vi "i2c_osd_cmd_write.vi"(5 "COM":bool, 7 "VISA name":refnum<visa-resource-name>, 9 "data":u8[](array[numeric]), 10 "byDataLen":u8, 11 "vdcmd_info_osd_t":T1) -> (3 "return":i32)   [LabVIEW 2016]
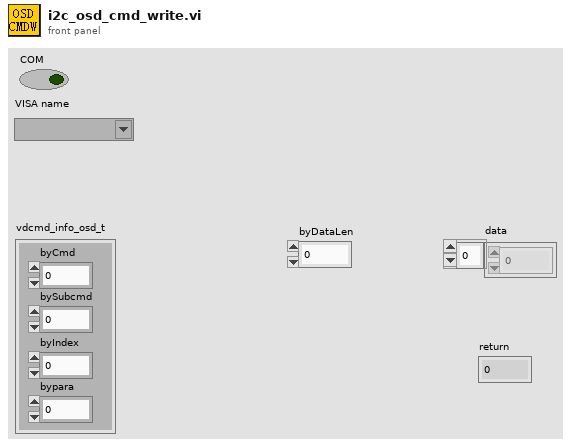
[diagram p1: front panel]
types:
  T1 = cluster{"byCmd":u8, "bySubcmd":u8, "byIndex":u8, "bypara":u8}
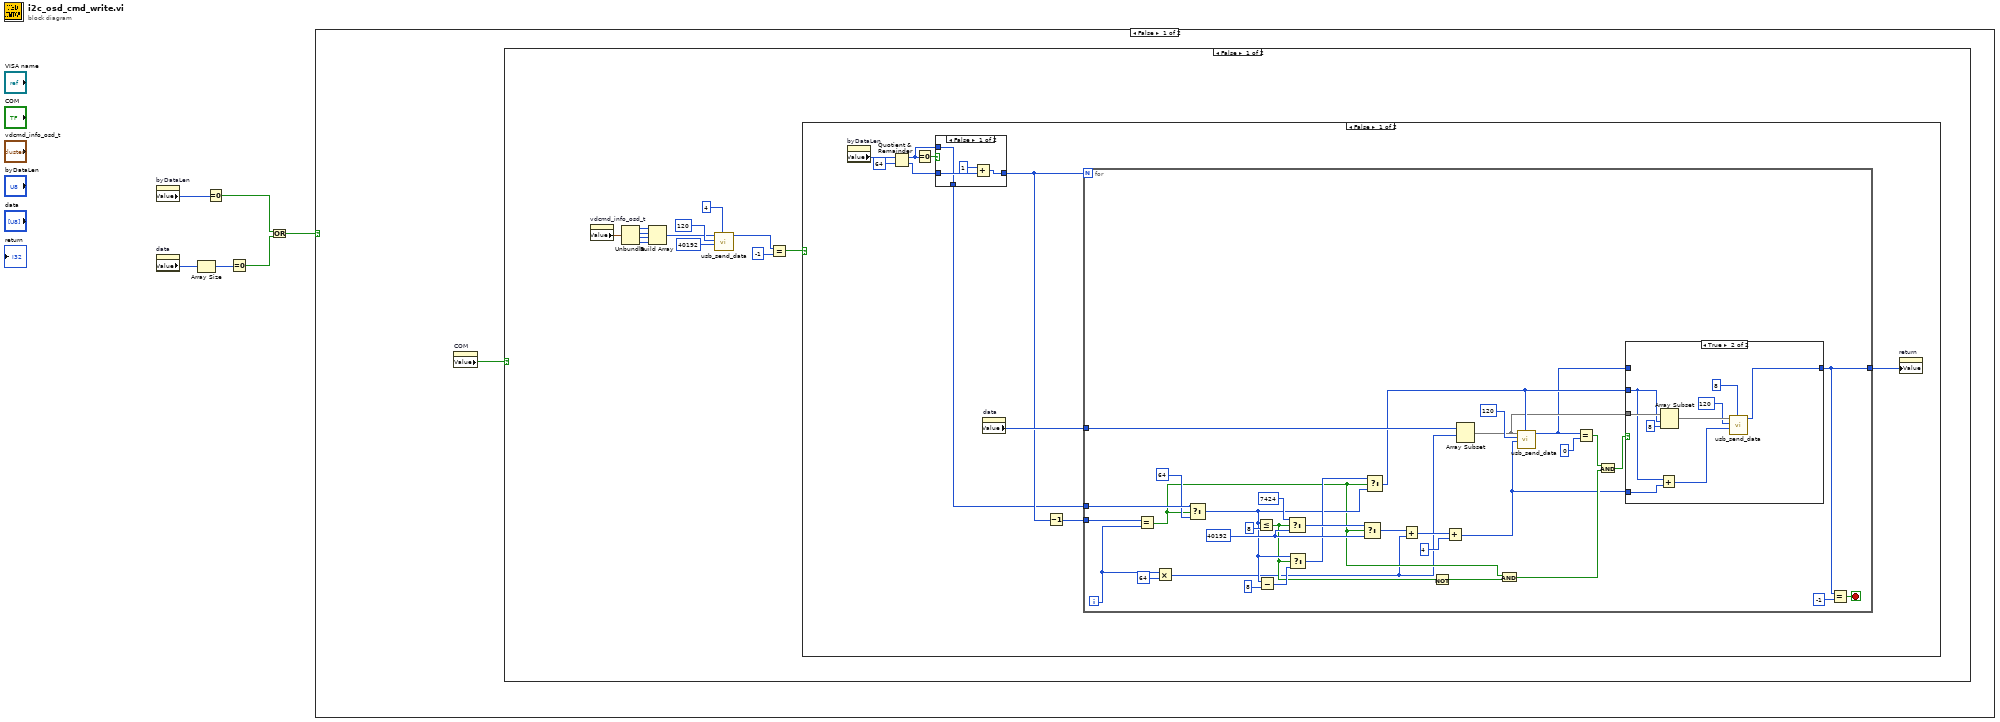
[diagram p0: block diagram]
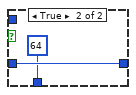
[diagram p3: hidden frame]
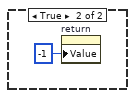
[diagram p4: hidden frame]
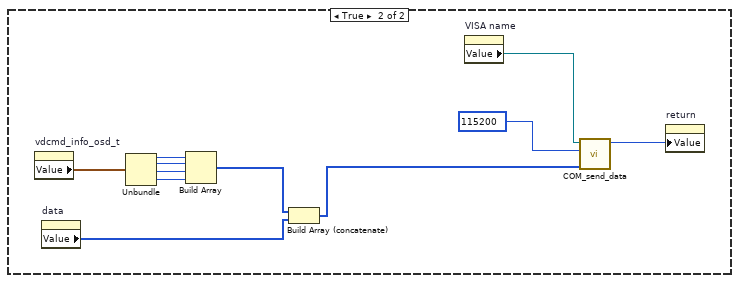
[diagram p5: hidden frame]
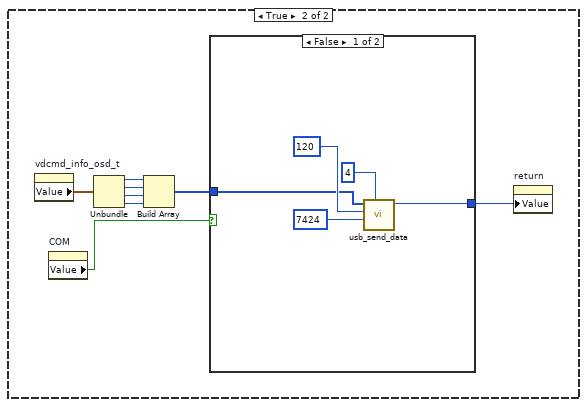
[diagram p6: hidden frame]
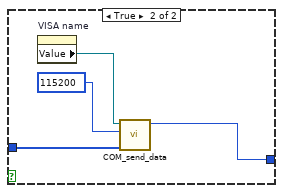
[diagram p7: hidden frame]
diagram:
  n1 = property on="byDataLen" class="DigNum (strict)"() -> ("Value"=w6:u8)  [unwired: 2 in, 2 out]
  n2 = property on="data" class="Arr (strict)"() -> ("Value"=w5:u8[])  [unwired: 2 in, 2 out]
  n3 = Array Size(array=w5) -> (size(s)=w4:i32)
  n4 = Equal To 0?(x=w6) -> (x = 0?=w2:bool)
  n5 = Equal To 0?(x=w4) -> (x = 0?=w3:bool)
  n6 = Or(x=w2, y=w3) -> (x .or. y?=w1:bool)
  n7 = case shown="False" w1 {
    frame False {
      n8 = property on="COM" class="Bool (strict)"() -> ("Value"=w7:bool)  [unwired: 2 in, 2 out]
      n9 = case shown="False" w7 {
        frame False {
          n10 = property on="vdcmd_info_osd_t" class="Clust (strict)"() -> ("Value"=w16:T1)  [unwired: 2 in, 2 out]
          n11 = Unbundle(w16) -> ("byCmd"=w15:u8, "bySubcmd"=w14:u8, "byIndex"=w13:u8, "bypara"=w12:u8)
          n12 = Build Array(w15, w14, w13, w12) -> (w11:u8[])
          n13 = call "usb_send_data.vi"("byVdCmdHeaderLen"=u16 4, "I2C_VD_BUFFER_RW"=u16 40192, "I2C_SLAVE_ID"=u8 120, "data"=w11) -> ("return"=w10:i32)  [unwired: 6 in, 1 out]
          n14 = Equal?(x=w10, y=-1) -> (x = y?=w8:bool)
          n15 = case shown="False" w8 {
            frame False {
              n16 = property on="byDataLen" class="DigNum (strict)"() -> ("Value"=w29:u8)  [unwired: 2 in, 2 out]
              n17 = Quotient & Remainder(x=w29, y=u8 64) -> (x-y*floor(x/y)=w23:u8, floor(x/y)=w26:u8)
              n18 = Equal To 0?(x=w23) -> (x = 0?=w27:bool)
              n19 = case shown="False" w27 {
                tunnel: w26 -> [w76 w78]
                tunnel: [w75 w78] -> w24
                tunnel: w23 -> [w73 _]
                tunnel: [w73 u8 64] -> w22
                frame False {
                  n20 = Add(x=u8 1, y=w76) -> (x+y=w75:u8)
                }
                frame True {
                }
              }
              n21 = property on="data" class="Arr (strict)"() -> ("Value"=w25:u8[])  [unwired: 2 in, 2 out]
              n22 = Decrement(x=w24) -> (x-1=w21:u8)
              n23 = for {
                N: w24 -> [_]
                tunnel: w25 -> [w60]
                tunnel: w21 -> [w62]
                tunnel: w22 -> [w58]
                tunnel: [w31] -> w20
                i -> [w59]
                stop <- w32 stop-if-true
                w47 = u16 40192 ("y")
                n24 = Equal?(x=w62, y=w59) -> (x = y?=w42:bool)
                n25 = Multiply(x=w59, y=64) -> (x*y=w30:i32)
                n26 = Select(t=w58, s=w42, f=u8 64) -> (s? t:f=w45:u8)
                n27 = Less Or Equal?(x=w45, y=u8 8) -> (x <= y?=w43:bool)
                n28 = Subtract(x=w45, y=u8 8) -> (x-y=w53:u8)
                n29 = Select(t=u16 7424 ("y"), s=w43, f=w47) -> (s? t:f=w48:u16)
                n30 = Select(t=w45, s=w43, f=w53) -> (s? t:f=w46:u8)
                n31 = Select(t=w48, s=w42, f=w47) -> (s? t:f=w49:u16)
                n32 = Select(t=w46, s=w42, f=w45) -> (s? t:f=w38:u8)
                n33 = Add(x=w49, y=w30) -> (x+y=w52:i32)
                n34 = Not(x=w43) -> (.not. x?=w41:bool)
                n35 = Add(x=w52, y=u16 4) -> (x+y=w36:i32)
                n36 = Array Subset(array=w60, index=w30) -> (w37:u8[])  [unwired: 1 in]
                n37 = And(x=w42, y=w41) -> (x .and. y?=w40:bool)
                n38 = call "usb_send_data.vi"("byVdCmdHeaderLen"=w38, "I2C_VD_BUFFER_RW"=w36, "I2C_SLAVE_ID"=u8 120, "data"=w37) -> ("return"=w34:i32)  [unwired: 6 in, 1 out]
                n39 = Equal?(x=w34, y=0) -> (x = y?=w35:bool)
                n40 = And(x=w35, y=w40) -> (x .and. y?=w39:bool)
                n41 = case shown="True" w39 {
                  tunnel: w38 -> [_ w67]
                  tunnel: w37 -> [_ w72]
                  tunnel: w36 -> [_ w68]
                  tunnel: w34 -> [w63 _]
                  tunnel: [w63 w65] -> w31
                  frame False {
                  }
                  frame True {
                    n42 = Add(x=w67, y=w68) -> (x+y=w66:i32)
                    n43 = Array Subset(array=w72, index=w67, length=8) -> (w70:u8[])
                    n44 = call "usb_send_data.vi"("byVdCmdHeaderLen"=u16 8, "I2C_VD_BUFFER_RW"=w66, "I2C_SLAVE_ID"=u8 120, "data"=w70) -> ("return"=w65:i32)  [unwired: 6 in, 1 out]
                  }
                }
                n45 = Equal?(x=w31, y=-1) -> (x = y?=w32:bool)
              }
              n46 = property on="return" class="DigNum (strict)"("Value"=w20) -> ()  [unwired: 2 in, 2 out]
            }
            frame True {
              n47 = property on="return" class="DigNum (strict)"("Value"=-1 ("return")) -> ()  [unwired: 2 in, 2 out]
            }
          }
        }
        frame True {
          n48 = property on="vdcmd_info_osd_t" class="Clust (strict)"() -> ("Value"=w88:T1)  [unwired: 2 in, 2 out]
          n49 = property on="data" class="Arr (strict)"() -> ("Value"=w82:u8[])  [unwired: 2 in, 2 out]
          n50 = Unbundle(w88) -> ("byCmd"=w87:u8, "bySubcmd"=w86:u8, "byIndex"=w85:u8, "bypara"=w84:u8)
          n51 = Build Array(w87, w86, w85, w84) -> (w83:u8[])
          n52 = Build Array (concatenate)(w83, w82) -> (w81:u8[])
          n53 = property on="VISA name" class="VISAName"() -> ("Value"=w90:refnum<visa-resource-name>)  [unwired: 2 in, 2 out]
          n54 = call "COM_send_data.vi"("data"=w81, "baud rate (9600)"=u32 115200, "VISA name"=w90) -> ("return"=w80:i32)  [unwired: 8 in]
          n55 = property on="return" class="DigNum (strict)"("Value"=w80) -> ()  [unwired: 2 in, 2 out]
        }
      }
    }
    frame True {
      n56 = property on="vdcmd_info_osd_t" class="Clust (strict)"() -> ("Value"=w98:T1)  [unwired: 2 in, 2 out]
      n57 = property on="COM" class="Bool (strict)"() -> ("Value"=w91:bool)  [unwired: 2 in, 2 out]
      n58 = Unbundle(w98) -> ("byCmd"=w97:u8, "bySubcmd"=w96:u8, "byIndex"=w95:u8, "bypara"=w94:u8)
      n59 = Build Array(w97, w96, w95, w94) -> (w93:u8[])
      n60 = case shown="False" w91 {
        tunnel: w93 -> [w100 w107]
        tunnel: [w99 w104] -> w92
        frame False {
          n61 = call "usb_send_data.vi"("byVdCmdHeaderLen"=u16 4, "I2C_VD_BUFFER_RW"=u16 7424, "I2C_SLAVE_ID"=u8 120, "data"=w100) -> ("return"=w99:i32)  [unwired: 6 in, 1 out]
        }
        frame True {
          n62 = property on="VISA name" class="VISAName"() -> ("Value"=w105:refnum<visa-resource-name>)  [unwired: 2 in, 2 out]
          n63 = call "COM_send_data.vi"("data"=w107, "baud rate (9600)"=u32 115200, "VISA name"=w105) -> ("return"=w104:i32)  [unwired: 8 in]
        }
      }
      n64 = property on="return" class="DigNum (strict)"("Value"=w92) -> ()  [unwired: 2 in, 2 out]
    }
  }
